vi "Delay.vi"(1 "Time Delay":dbl) -> (0 "Delay Not Reached":bool)   [LabVIEW 2015]
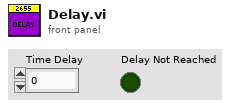
[diagram p1: front panel]
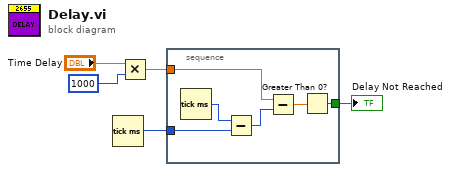
[diagram p0: block diagram]
diagram:
  n1 = Tick Count (ms)() -> (millisecond timer value=w5:u32)
  n2 = Multiply(x="Time Delay", y=1000) -> (x*y=w4:dbl)
  n3 = stacked-sequence {
    tunnel: w5 -> [w11]
    tunnel: w4 -> [w10]
    tunnel: [w6] -> w1
    frame #0 {
      n4 = Tick Count (ms)() -> (millisecond timer value=w8:u32)
      n5 = Subtract(x=w8, y=w11) -> (x-y=w9:u32)
      n6 = Subtract(x=w10, y=w9) -> (x-y=w7:dbl)
      n7 = Greater Than 0?(x=w7) -> (x > 0?=w6:bool)
    }
  }
  "Delay Not Reached" <- w1
